vi "submanuelebediening.vi"(5 "rechts draaien":bool, 6 "voorwaarts":bool, 7 "links draaien":bool, 10 "achterwaarts":bool) -> ()   [LabVIEW 2019]
uses:
  <vilib>/myRIO/Common/Instrument Driver Framework/Utilities/typedefs/Analog Scaling Constants.ctl
  <vilib>/myRIO/Common/Instrument Driver Framework/Utilities/typedefs/Analog Scaling Constants List.ctl
  <vilib>/myRIO/Common/Instrument Driver Framework/myRIO v1.0/AO/typedefs/AO Channels Enum.ctl
  <vilib>/myRIO/Common/Instrument Driver Framework/myRIO v1.0/AO/typedefs/AO Channels List.ctl
  <vilib>/myRIO/Common/Instrument Driver Framework/Utilities/typedefs/Generic FPGA Reference.ctl
  <vilib>/myRIO/Common/Instrument Driver Framework/Utilities/typedefs/myRIO v1.0 Reference.ctl
  <vilib>/myRIO/Common/Instrument Driver Framework/Utilities/typedefs/Hardware Version Enum.ctl
  <vilib>/myRIO/Common/Instrument Driver Framework/Utilities/typedefs/myRIO Generic Hardware Reference.ctl
  <vilib>/myRIO/Instrument Drivers/Onboard IO/AO/typedefs/AO Reference.ctl
  <vilib>/myRIO/Instrument Drivers/Onboard IO/AO/AO.lvlib
  <vilib>/myRIO/Instrument Drivers/Onboard IO/AO/vis/Write.vi
  <vilib>/userDefined/High Color/nirio_resource_hc.ctl
  <vilib>/myRIO/Common/Instrument Driver Framework/myRIO v1.0/AO/vis/myRIO v1.1 Open AO.vi
  <vilib>/myRIO/Instrument Drivers/Onboard IO/AO/vis/myRIO AO Open.xnode
  <vilib>/myRIO/Common/Instrument Driver Framework/Utilities/vis/Is FPGA Ref Available.vi
  <vilib>/myRIO/Express VI/Onboard IO/AO/AO Express VI.xnode
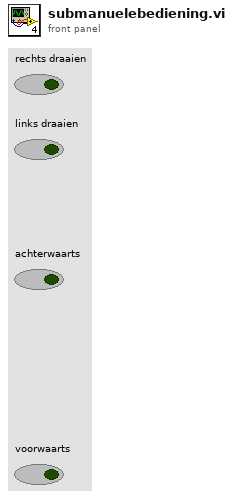
[diagram p1: front panel]
types:
  T1 = typedef "AO.lvlib/AO Reference.ctl" = cluster{"myRIO Reference":T2, "AO Channel List":T6, "AO Scaling Constant List":T8}
  T2 = typedef "myRIO Generic Hardware Reference.ctl" = cluster{"myRIO Model":T3, "myRIO Hardware Reference":T4}
  T3 = typedef "Hardware Version Enum.ctl" = enum16{"Unknown", "myRIO-1900", "myRIO-1950", "roboRIO", "NI ELVIS RIO CM", "ELVIS III"}
  T4 = typedef "myRIO v1.0 Reference.ctl" = cluster{"Generic FPGA Reference":T5, "Allow multiple opens":bool}
  T5 = typedef "Generic FPGA Reference.ctl" = refnum<k20>
  T6 = typedef "AO Channels List.ctl" = T7[]
  T7 = typedef "AO Channels Enum.ctl" = enum16{"Not Connected", "AudioOut/Left", "AudioOut/Right", "C/AO0", "C/AO1", "A/AO0", "A/AO1", "B/AO0", "B/AO1"}
  T8 = typedef "Analog Scaling Constants List.ctl" = T9[]
  T9 = typedef "Analog Scaling Constants.ctl" = cluster{"LSB Weight (Volts)":dbl, "Offset (Volts)":dbl, "Signed?":bool}
  T10 = typedef "nirio_resource_hc.ctl" = tag
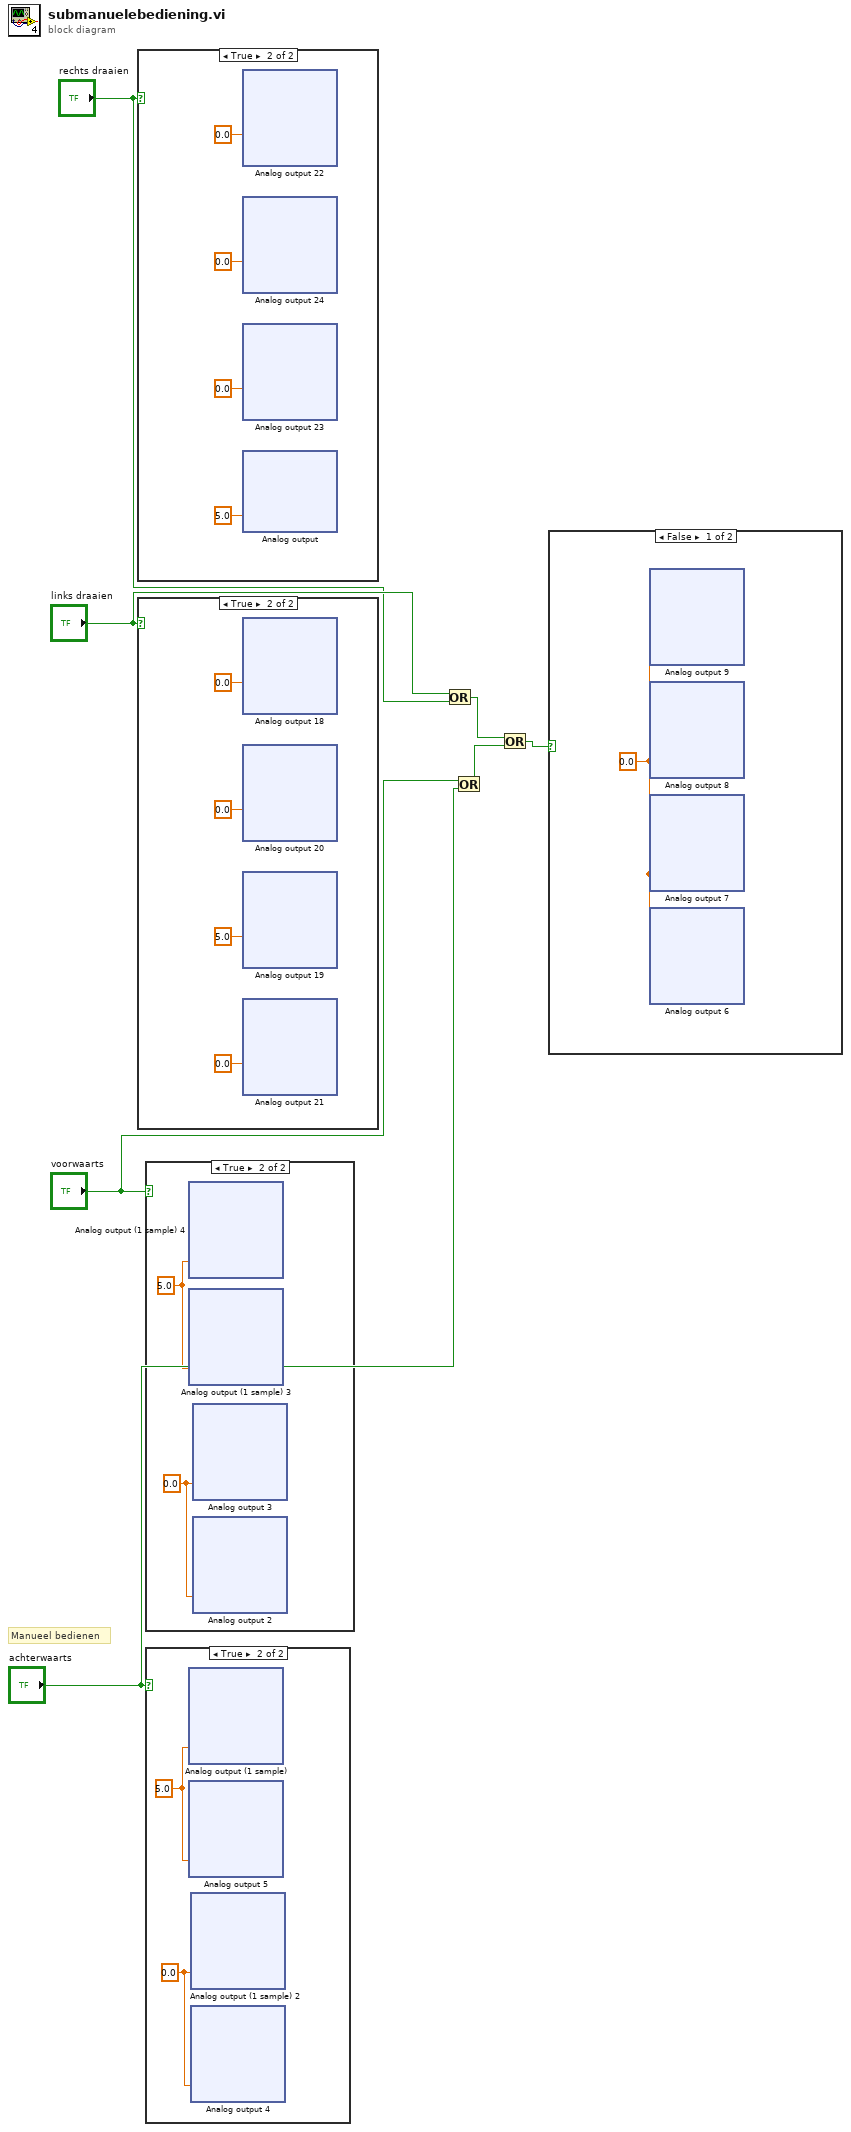
[diagram p0: block diagram]
diagram:
  # "Manueel bedienen"
  n1 = case shown="True" "rechts draaien" {
    frame False {
    }
    frame True {
      n2 = xnode "Analog output 22"("B/AO1 (Pin 4)"=0.0) -> ()  [unwired: 1 in, 1 out]
      n3 = xnode "Analog output 24"("A/AO1 (Pin 4)"=0.0) -> ()  [unwired: 1 in, 1 out]
      n4 = xnode "Analog output 23"("B/AO0 (Pin 2)"=0.0) -> ()  [unwired: 1 in, 1 out]
      n5 = xnode "Analog output"("A/AO0 (Pin 2)"=5.0) -> ()  [unwired: 1 in, 1 out]
    }
  }
  n6 = case shown="True" "links draaien" {
    frame False {
    }
    frame True {
      n7 = xnode "Analog output 18"("B/AO1 (Pin 4)"=0.0) -> ()  [unwired: 1 in, 1 out]
      n8 = xnode "Analog output 20"("A/AO1 (Pin 4)"=0.0) -> ()  [unwired: 1 in, 1 out]
      n9 = xnode "Analog output 19"("B/AO0 (Pin 2)"=5.0) -> ()  [unwired: 1 in, 1 out]
      n10 = xnode "Analog output 21"("A/AO0 (Pin 2)"=0.0) -> ()  [unwired: 1 in, 1 out]
    }
  }
  n11 = case shown="True" "voorwaarts" {
    frame False {
    }
    frame True {
      w312 = 5.0
      w313 = 0.0
      n12 = xnode "Analog output (1 sample) 4"("A/AO0 (Pin 2)"=w312) -> ()  [unwired: 1 in, 1 out]
      n13 = xnode "Analog output (1 sample) 3"("B/AO0 (Pin 2)"=w312) -> ()  [unwired: 1 in, 1 out]
      n14 = xnode "Analog output 3"("A/AO1 (Pin 4)"=w313) -> ()  [unwired: 1 in, 1 out]
      n15 = xnode "Analog output 2"("B/AO1 (Pin 4)"=w313) -> ()  [unwired: 1 in, 1 out]
    }
  }
  n16 = case shown="True" "achterwaarts" {
    frame False {
    }
    frame True {
      w462 = 5.0
      w463 = 0.0
      n17 = xnode "Analog output (1 sample)"("A/AO1 (Pin 4)"=w462) -> ()  [unwired: 1 in, 1 out]
      n18 = xnode "Analog output 5"("B/AO1 (Pin 4)"=w462) -> ()  [unwired: 1 in, 1 out]
      n19 = xnode "Analog output (1 sample) 2"("A/AO0 (Pin 2)"=w463) -> ()  [unwired: 1 in, 1 out]
      n20 = xnode "Analog output 4"("B/AO0 (Pin 2)"=w463) -> ()  [unwired: 1 in, 1 out]
    }
  }
  n21 = Or(x="links draaien", y="rechts draaien") -> (x .or. y?=w6:bool)
  n22 = Or(x="voorwaarts", y="achterwaarts") -> (x .or. y?=w7:bool)
  n23 = Or(x=w6, y=w7) -> (x .or. y?=w5:bool)
  n24 = case shown="False" w5 {
    frame False {
      w612 = 0.0
      n25 = xnode "Analog output 9"("A/AO0 (Pin 2)"=w612) -> ()  [unwired: 1 in, 1 out]
      n26 = xnode "Analog output 8"("A/AO1 (Pin 4)"=w612) -> ()  [unwired: 1 in, 1 out]
      n27 = xnode "Analog output 7"("B/AO0 (Pin 2)"=w612) -> ()  [unwired: 1 in, 1 out]
      n28 = xnode "Analog output 6"("B/AO1 (Pin 4)"=w612) -> ()  [unwired: 1 in, 1 out]
    }
    frame True {
    }
  }
